vi "venier pH read v1_0.vi"() -> (0 "mean":dbl format="%0.2f")   [LabVIEW 2012]
uses:
  <vilib>/Analysis/baseanly.llb/Mean (DBL).vi
  <vilib>/Analysis/NI_AALBase.lvlib
panel:
  out "error":i32
  out "Temp/Link 1: Stored Data Array":dbl[](array[numeric])
  in  "Length of Experiment (sec)":dbl=0.1
  in  "Sample Rate (samples/sec)":dbl=10.0 min=0.0 max=48000.0 step=0.1 format="%#.0f"
  # "The is a striped down version of \"go test fast\" so it can be wired to be a subVI.\n(! The Go drivers not very robust? Or is it Windows? Broke when we moved the VI. If so, quit Labview and relaunch.)"
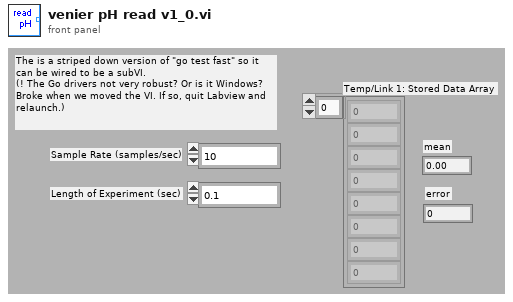
[diagram p1: front panel]
types:
  T1 = typedef "GO_Setup Parameters Cluster.ctl" = cluster{"Go! Device Handle Array":i32[], "Comm port (LabPro only)":i32, "Config":T2}
  T2 = typedef "GO_Config Cluster.ctl" = cluster{"Sensor Info Array":T3[], "Y min 1":dbl, "Y min 2":dbl, "Y min 3":dbl, "Y min 4":dbl, "Y max 1":dbl, "Y max 2":dbl, "Y max 3":dbl, "Y max 4":dbl, "Pos Y min":dbl, "Vel Y min":dbl, "Accel Y min":dbl, "Pos Y max":dbl, "Vel Y max":dbl, "Accel Y max":dbl, "X min":dbl, "X max":dbl, "sample rate (sample/sec)":dbl, "sample time (sec/sample)":dbl, "# of samples":u32, "Repeat?":bool, "Active Channel Array":bool[], "MD Active Ch Array":bool[], "# active probes":u32, "TrigType":T4, "TrigChan":i32, "TrigThresh":dbl, "Pre-Store (%)":i32, "Pre-store (#samp)":u32, "Short Sensor Name":string[], "Product ID Array":u8[]}
  T3 = typedef "GO_Sensor Info Cluster.ctl" = cluster{"Long Name":string, "Active CalPage":u8, "Calpage Coefficients":cluster{"K0":sgl, "K1":sgl, "K2":sgl, "Units":string}[], "Equation Type":u8, "Operation Type":u8, "Num Valid Cal Pages":u8}
  T4 = typedef "GO_TrigType Enum.ctl" = enum16{"No Trigger", "Analog Trigger - Rising", "Analog Trigger - Falling"}
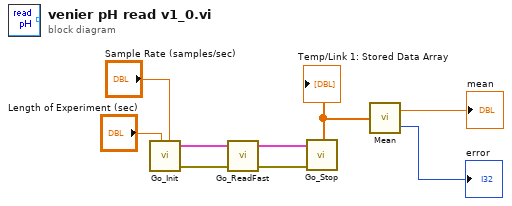
[diagram p0: block diagram]
diagram:
  n1 = call <vilib>:"Go_Init.vi"("Length of Experiment (sec)"="Length of Experiment (sec)", "Sample Rate (samples/sec)"="Sample Rate (samples/sec)") -> ("Setup Parameters"=w7:T1, "error out"=w6:errorcluster)  [unwired: 4 in, 2 out]
  n2 = call <vilib>:"Go_ReadFast.vi"("Parameters"=w7, "error in"=w6) -> ("Parameters"=w5:T1, "error out"=w4:errorcluster)  [unwired: 2 in, 4 out]
  n3 = call <vilib>:"Go_Stop.vi"("Parameters"=w5, "error in"=w4) -> ("Temp/Link 1: Stored Data Array"=w3:dbl[])  [unwired: 3 in, 4 out]
  "Temp/Link 1: Stored Data Array" <- w3
  n4 = call-poly <vilib>:"Mean.vi"("X"=w3) -> ("mean"=→"mean":dbl, "error"=→"error":i32)
